vi "shutter1.vi"() -> ()   [LabVIEW 2013]
panel:
  in  "stop":bool
  in  "Shutter Position":bool
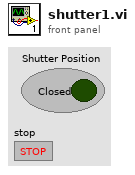
[diagram p1: front panel]
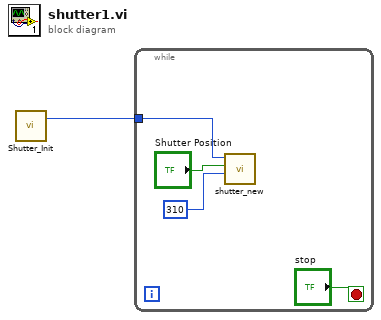
[diagram p0: block diagram]
diagram:
  n1 = call "Shutter_Init.vi"() -> ("ObjectPtr"=w1:i32)  [unwired: 2 in, 1 out]
  n2 = while {
    tunnel: w1 -> [w4]
    stop <- "stop" stop-if-true
    n3 = call "shutter_new.vi"("ShutterID"=310, "Shutter Position"="Shutter Position", "ObjectPtr"=w4) -> ()  [unwired: 1 in, 1 out]
  }
